vi "Add with Carry.vi"(10 "Input 2":u8 format="%08b", 11 "Input 1":u8 format="%08b") -> (2 "Carry":bool, 3 "Output":u8 format="%08b")   [LabVIEW 2025, in "TD4.lvclass"]
uses:
  TD4.lvclass
  TD4.lvclass/TD4.ctl
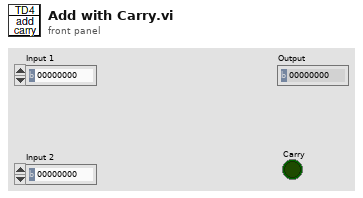
[diagram p1: front panel]
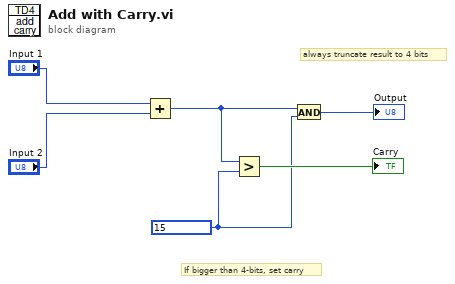
[diagram p0: block diagram]
diagram:
  w2 = u8 15
  # "always truncate result to 4 bits"
  # "If bigger than 4-bits, set carry"
  n1 = Add(x="Input 1", y="Input 2") -> (x+y=w3:u8)
  n2 = Greater?(x=w3, y=w2) -> (0:→"Carry":bool)
  n3 = And(x=w3, y=w2) -> (x .and. y?=→"Output":u8)
